vi "Add Entries.vi"(8 "error in":errorcluster, 10 "Item Data":refnum<class "Item.lvclass">[](array[class]), 11 "Tree Map in":refnum<class "Project Tree Map.lvclass">) -> (0 "error out":errorcluster, 3 "Tree Map out":refnum<class "Project Tree Map.lvclass">)   [LabVIEW 2020, in "VI Properties Editor.lvlib" / "Project Tree Map.lvclass"]
doc: "Adds all entries to the tree map."
uses:
  Project Tree Map.lvclass
  Item/Item.lvclass
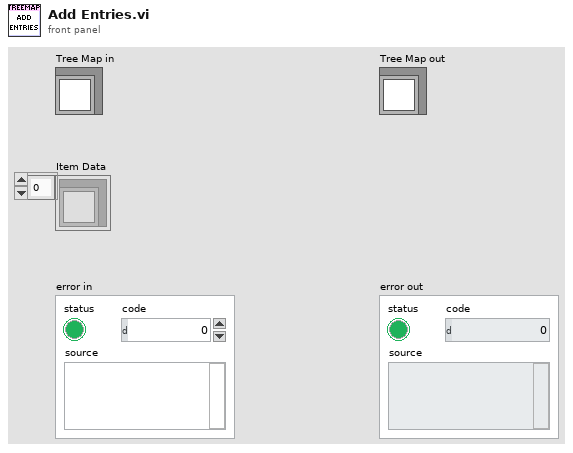
[diagram p1: front panel]
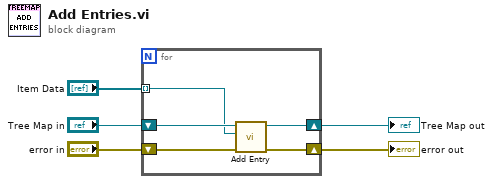
[diagram p0: block diagram]
diagram:
  n1 = for {
    tunnel: "Item Data" -> [w6] mode=indexing
    shift-right: [w8] -> w2
    shift-left: "Tree Map in" -> [w10]
    shift-right: [w7] -> w1
    shift-left: "error in" -> [w9]
    n2 = call "Add Entry.vi"("error in"=w9, "Item"=w6, "Tree Map in"=w10) -> ("error out"=w7:errorcluster, "Tree Map out"=w8:refnum<class "Project Tree Map.lvclass">)  [unwired: 7 in]
  }
  "Tree Map out" <- w2
  "error out" <- w1
